vi "HPWH Check End Of Draw Full Credit.vi"(5 "Upper Most Element":T1=enum."Lower Element", 7 "Draw_Start":dbl, 8 "error in (no error)":errorcluster, 11 "Test Start to End":string[][](array[string])) -> (0 "error out":errorcluster, 3 "Cutout Time (Seconds)":dbl)   [LabVIEW 2023]
uses:
  Type Definitions/Upper Most Element.ctl
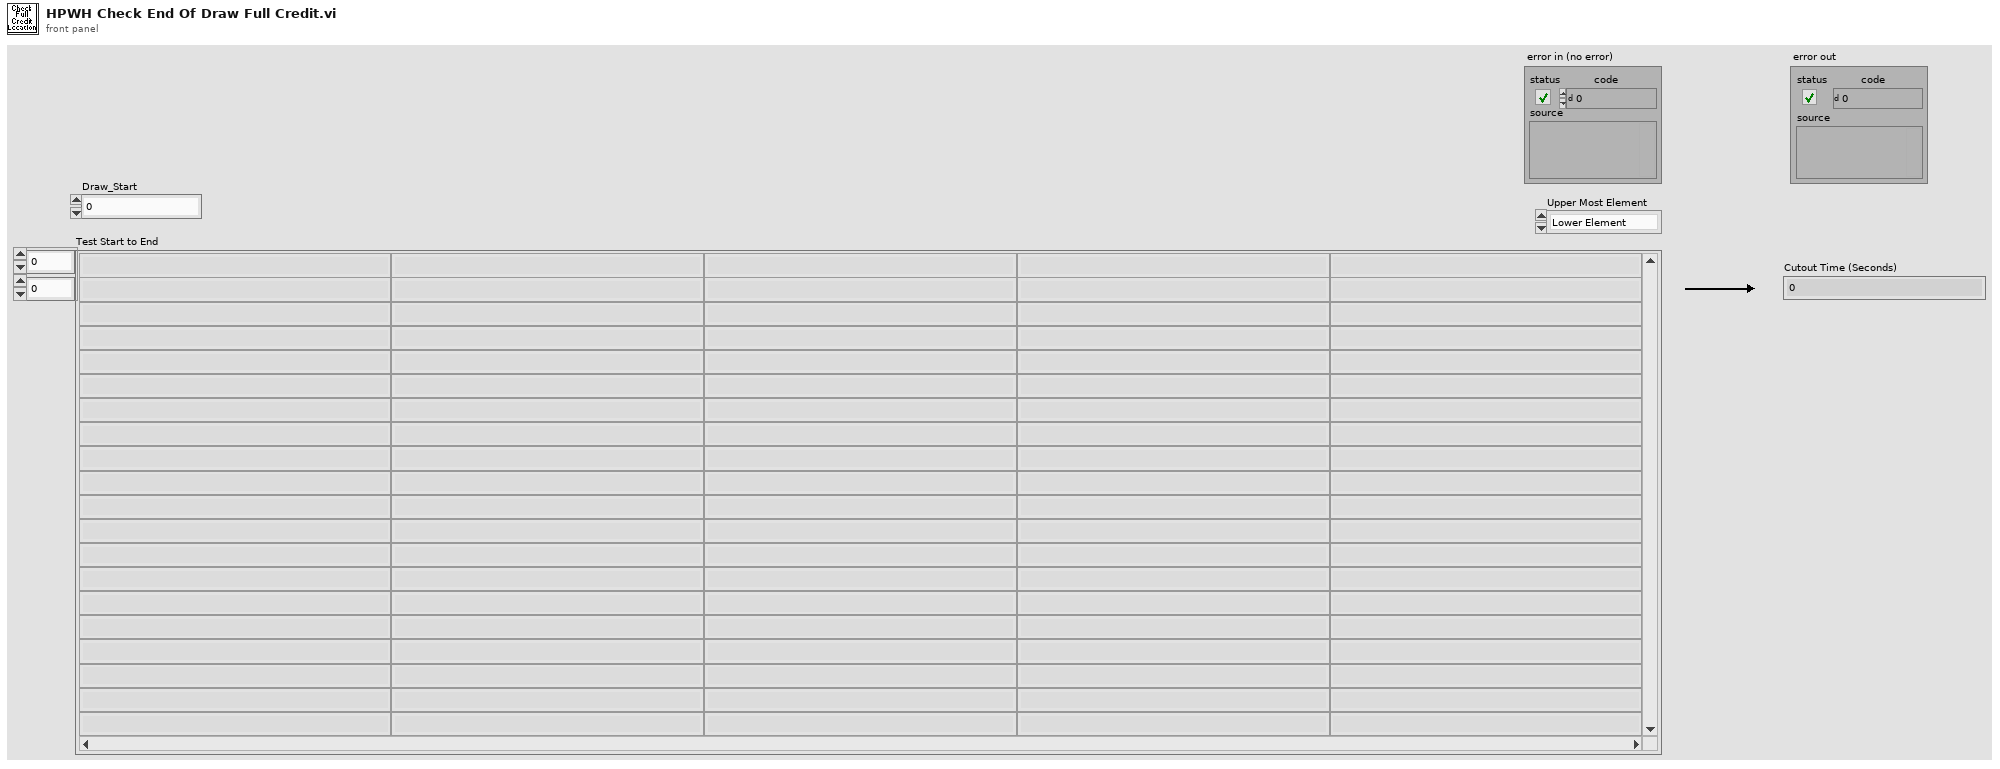
[diagram p1: front panel]
types:
  T1 = typedef "Upper Most Element.ctl" = enum16{"Compressor", "Lower Element", "Upper Element"}
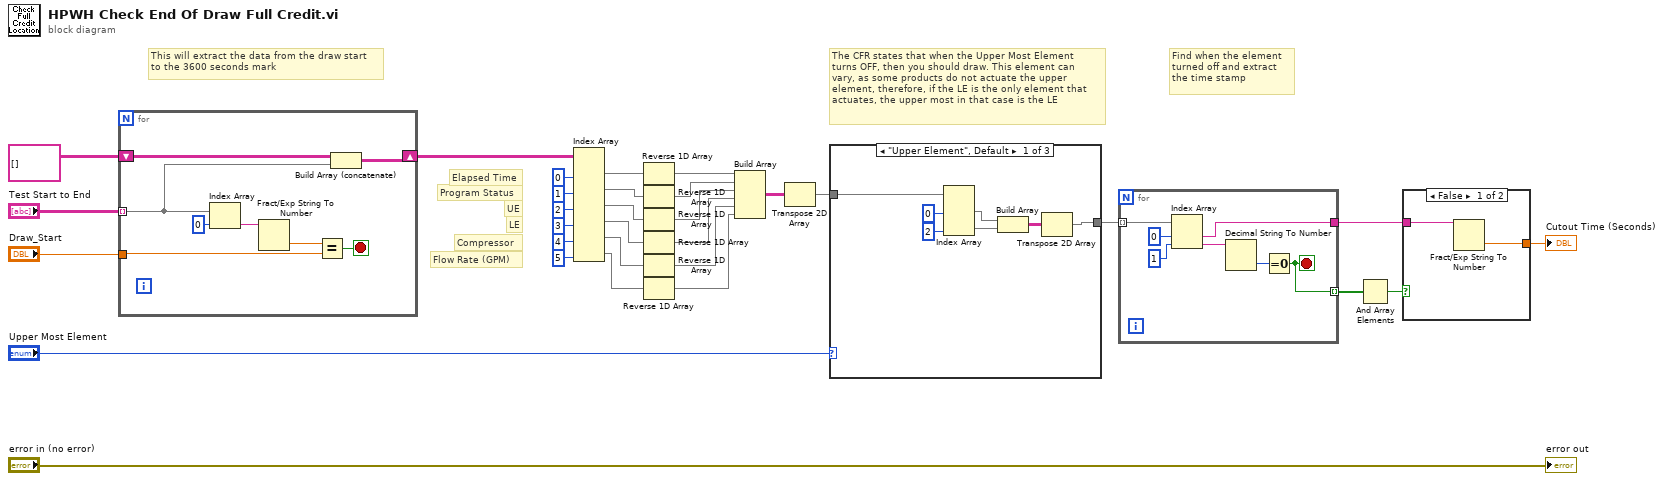
[diagram p0: block diagram]
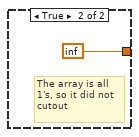
[diagram p2: hidden frame]
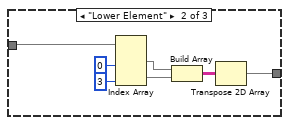
[diagram p3: hidden frame]
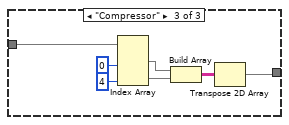
[diagram p4: hidden frame]
diagram:
  # "Flow Rate (GPM)"
  # "Compressor"
  # "LE"
  # "UE"
  # "Program Status"
  # "Elapsed Time"
  # "Find when the element\nturned off and extract\nthe time stamp"
  # "The CFR states that when the Upper Most Element\nturns OFF, then you should draw. This element can\nvary, as some products do not actuate the upper\nelement, therefore, if the LE is the only element that\nactuates, the upper most in that case is the LE"
  # "This will extract the data from the draw start\nto the 3600 seconds mark"
  n1 = for {
    tunnel: "Test Start to End" -> [w33] mode=indexing
    tunnel: "Draw_Start" -> [w35]
    shift-right: [w32] -> w15
    shift-left: string[][] [] -> [w34]
    stop <- w38 stop-if-true
    n2 = Index Array(array=w33, index=0) -> (element=w37:string)
    n3 = Fract/Exp String To Number(string=w37) -> (number=w36:dbl)  [unwired: 3 in, 1 out]
    n4 = Equal?(x=w36, y=w35) -> (x = y?=w38:bool)
    n5 = Build Array (concatenate)(w34, w33) -> (w32:string[][])
  }
  n6 = Index Array(array=w15, index (col) #1=0 ("disabled index (col)"), index (col) #2=1 ("index (col)"), index (col) #3=2 ("index (col)"), index (col) #4=3 ("index (col)"), index (col) #5=4 ("index (col)"), index (col) #6=5 ("index (col)")) -> (element #1=w16:string[], element #2=w17:string[], element #3=w21:string[], element #4=w22:string[], element #5=w23:string[], element #6=w27:string[])  [unwired: 6 in]
  n7 = Reverse 1D Array(array=w16) -> (reversed array=w18:string[])
  n8 = Reverse 1D Array(array=w17) -> (reversed array=w19:string[])
  n9 = Reverse 1D Array(array=w21) -> (reversed array=w24:string[])
  n10 = Reverse 1D Array(array=w22) -> (reversed array=w25:string[])
  n11 = Reverse 1D Array(array=w23) -> (reversed array=w26:string[])
  n12 = Reverse 1D Array(array=w27) -> (reversed array=w28:string[])
  n13 = Build Array(w18, w19, w24, w25, w26, w28) -> (w20:string[][])
  n14 = Transpose 2D Array(2D array=w20) -> (transposed array=w8:string[][])
  n15 = case shown="\"Upper Element\", Default" "Upper Most Element" {
    tunnel: w8 -> [w46 w53 w60]
    tunnel: [w40 w47 w54] -> w6
    frame "Upper Element", Default {
      n16 = Index Array(array=w46, index (col) #1=0 ("disabled index (col)"), index (col) #2=2 ("disabled index (col)")) -> (element #1=w42:string[], element #2=w41:string[])  [unwired: 2 in]
      n17 = Build Array(w42, w41) -> (w43:string[][])
      n18 = Transpose 2D Array(2D array=w43) -> (transposed array=w40:string[][])
    }
    frame "Lower Element" {
      n19 = Index Array(array=w53, index (col) #1=0 ("disabled index (col)"), index (col) #2=3 ("disabled index (col)")) -> (element #1=w49:string[], element #2=w48:string[])  [unwired: 2 in]
      n20 = Build Array(w49, w48) -> (w50:string[][])
      n21 = Transpose 2D Array(2D array=w50) -> (transposed array=w47:string[][])
    }
    frame "Compressor" {
      n22 = Index Array(array=w60, index (col) #1=0 ("disabled index (col)"), index (col) #2=4 ("disabled index (col)")) -> (element #1=w57:string[], element #2=w56:string[])  [unwired: 2 in]
      n23 = Build Array(w57, w56) -> (w55:string[][])
      n24 = Transpose 2D Array(2D array=w55) -> (transposed array=w54:string[][])
    }
  }
  n25 = for {
    tunnel: w6 -> [w67] mode=indexing
    tunnel: [w62] -> w3
    tunnel: [w61] -> w5 mode=indexing
    stop <- w61 stop-if-true
    n26 = Index Array(array=w67, index #1=0 ("index"), index #2=1 ("index")) -> (element #1=w62:string, element #2=w64:string)
    n27 = Decimal String To Number(string=w64) -> (number=w63:i32)  [unwired: 2 in, 1 out]
    n28 = Equal To 0?(x=w63) -> (x = 0?=w61:bool)
  }
  n29 = And Array Elements(Boolean array=w5) -> (logical AND=w4:bool)
  n30 = case shown="False" w4 {
    tunnel: w3 -> [w69 _]
    tunnel: [w68 inf] -> w2
    frame False {
      n31 = Fract/Exp String To Number(string=w69) -> (number=w68:dbl)  [unwired: 3 in, 1 out]
    }
    frame True {
      # "The array is all\n1's, so it did not \ncutout"
    }
  }
  "Cutout Time (Seconds)" <- w2
  "error out" <- "error in (no error)"
